vi "add parameter indicies controls.vi"(8 "error in":errorcluster, 9 "Channels to create":T1[](array[typedef]), 10 "class path":path, 11 "Application in":refnum<vi>) -> (0 "error out":errorcluster, 2 "Disable Channel Group?":bool[](array[boolean]))   [LabVIEW 2013, in "FixedChannelTBModuleDecideFeatures.lvclass"]
uses:
  FixedChannelTBModuleDecideFeatures.lvclass
  channel configuration.ctl
  <vilib>/NI/Tag Bus Module Framework/channel/channel classification.ctl
  <vilib>/NI/Tag Bus/tag/Data Type.ctl
  <vilib>/Utility/traverseref.llb/TRef TravTarget.ctl
  <vilib>/NI/Tag Bus Module Framework/channel/TBM channel.lvclass
  <vilib>/Utility/traverseref.llb/VI Scripting - Traverse.lvlib
  <vilib>/NI/Tag Bus/tag/tag descriptor.lvclass
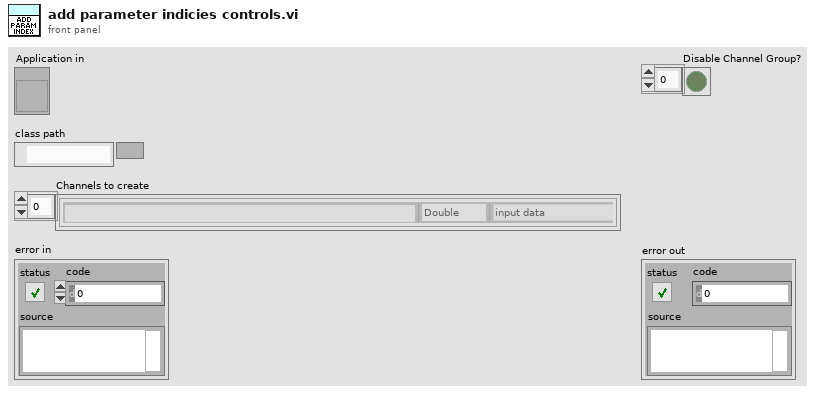
[diagram p1: front panel]
types:
  T1 = typedef "FixedChannelTBModuleDecideFeatures.lvclass/channel configuration.ctl" = cluster{"Name":string, "channel classification":T2, "data type":T3}
  T2 = typedef "TBM channel.lvclass/channel classification.ctl" = enum16{"input data", "output data", "processing parameter", "processing result"}
  T3 = typedef "tag bus.lvlib/tag descriptor.lvclass/Data Type.ctl" = enum16{"Double", "Single", "I64", "I32", "I16", "I8", "U64", "U32", "U16", "U8", "Boolean", "String", "Array of Double", "Array of Single", "Array of I64", "Array of I32", "Array of I16", "Array of I8", "Array of U64", "Array of U32", "Array of U16", "Array of U8", "Array of Boolean", "Array of String"}
  T4 = typedef "TRef TravTarget.ctl" = enum16{"FP", "BD", "Other"}
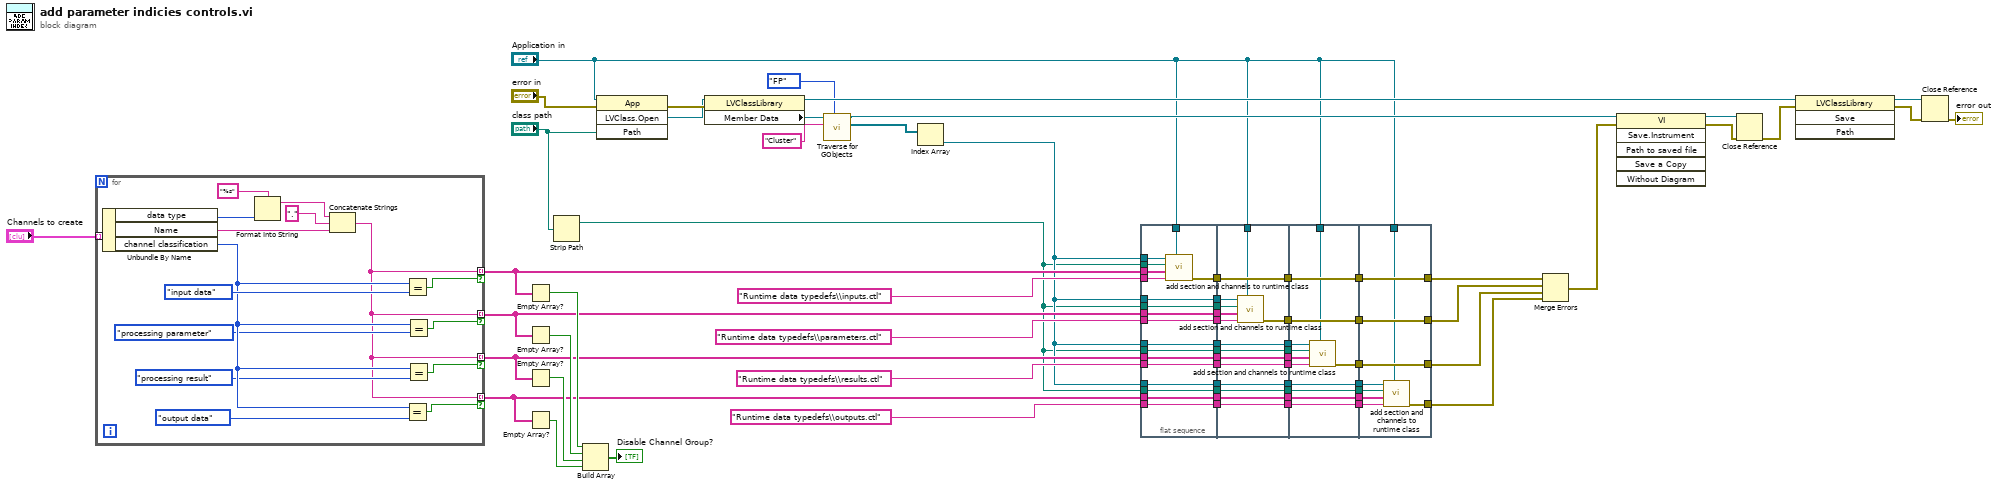
[diagram p0: block diagram]
diagram:
  n1 = for {
    tunnel: "Channels to create" -> [w84] mode=indexing
    tunnel: [w70] -> w51 mode=indexing if=w82
    tunnel: [w70] -> w47 mode=indexing if=w81
    tunnel: [w70] -> w37 mode=indexing if=w79
    tunnel: [w70] -> w25 mode=indexing if=w80
    n2 = Unbundle By Name(w84) -> ("data type"=w74:T3, "Name"=w72:string, "channel classification"=w78:T2)
    n3 = Format Into String(format string="%s", w74) -> (resulting string=w73:string)  [unwired: 2 in, 1 out]
    n4 = Concatenate Strings(w73, "." ("string"), w72) -> (w70:string)
    n5 = Equal?(x=w78, y=channel_classification."output data" ("x")) -> (x = y?=w80:bool)
    n6 = Equal?(x=w78, y=channel_classification."input data" ("x")) -> (x = y?=w82:bool)
    n7 = Equal?(x=w78, y=channel_classification."processing parameter" ("x")) -> (x = y?=w81:bool)
    n8 = Equal?(x=w78, y=channel_classification."processing result" ("x")) -> (x = y?=w79:bool)
  }
  n9 = Empty Array?(array=w51) -> (empty?=w56:bool)
  n10 = Empty Array?(array=w47) -> (empty?=w55:bool)
  n11 = Empty Array?(array=w37) -> (empty?=w54:bool)
  n12 = Empty Array?(array=w25) -> (empty?=w53:bool)
  n13 = Strip Path(path="class path") -> (stripped path=w26:path)  [unwired: 1 out]
  n14 = Build Array(w56, w55, w54, w53) -> (→"Disable Channel Group?":bool[])
  n15 = invoke class="App" method="LVClass.Open"(reference="Application in", error in="error in", "Path"="class path") -> (error out=w68:errorcluster, "LVClass.Open"=w2:refnum<vi>)  [unwired: 1 in, 2 out]
  n16 = property class="LVClassLibrary"(reference=w2, error in=w68) -> (reference out=w65:refnum<vi>, "Member Data"=w3:refnum<vi>)  [unwired: 1 out]
  n17 = call <vilib>:"Traverse for GObjects.vi"("Traverse Target"=TRef_TravTarget."FP", "Class Name"="Cluster", "VI Refnum"=w3) -> ("References"=w4:refnum<vi>[], "dup VI Refnum"=w7:refnum<vi>)  [unwired: 5 in, 2 out]
  n18 = Index Array(array=w4) -> (element=w30:refnum<vi>)  [unwired: 1 in]
  n19 = flat-sequence {
    tunnel: w51 -> [w102]
    tunnel: "Runtime data typedefs\\inputs.ctl" ("name or relative path") -> [w101]
    tunnel: w26 -> [w100]
    tunnel: w30 -> [w86]
    tunnel: w30 -> [w99]
    tunnel: [w99] -> w49
    tunnel: [w98] -> w48
    tunnel: w26 -> [w98]
    tunnel: w47 -> [w97]
    tunnel: [w97] -> w46
    tunnel: [w96] -> w45
    tunnel: "Runtime data typedefs\\parameters.ctl" ("name or relative path") -> [w96]
    tunnel: [w95] -> w42
    tunnel: w30 -> [w95]
    tunnel: [w94] -> w40
    tunnel: w26 -> [w94]
    tunnel: [w93] -> w38
    tunnel: w37 -> [w93]
    tunnel: "Runtime data typedefs\\results.ctl" ("name or relative path") -> [w92]
    tunnel: [w92] -> w34
    tunnel: [w91] -> w31
    tunnel: w30 -> [w91]
    tunnel: [w90] -> w27
    tunnel: w26 -> [w90]
    tunnel: w25 -> [w89]
    tunnel: [w89] -> w24
    tunnel: [w88] -> w19
    tunnel: "Runtime data typedefs\\outputs.ctl" ("name or relative path") -> [w88]
    tunnel: [w87] -> w14
    tunnel: "Application in" -> [w85]
    tunnel: w49 -> [w117]
    tunnel: w48 -> [w116]
    tunnel: w46 -> [w115]
    tunnel: w45 -> [w114]
    tunnel: [w113] -> w43
    tunnel: w42 -> [w113]
    tunnel: [w112] -> w41
    tunnel: w40 -> [w112]
    tunnel: [w111] -> w39
    tunnel: w38 -> [w111]
    tunnel: [w110] -> w35
    tunnel: w34 -> [w110]
    tunnel: [w109] -> w32
    tunnel: w31 -> [w109]
    tunnel: [w108] -> w28
    tunnel: w27 -> [w108]
    tunnel: w24 -> [w107]
    tunnel: [w107] -> w23
    tunnel: [w106] -> w20
    tunnel: w19 -> [w106]
    tunnel: [w105] -> w15
    tunnel: w14 -> [w105]
    tunnel: [w104] -> w12
    tunnel: "Application in" -> [w103]
    tunnel: w43 -> [w129]
    tunnel: w41 -> [w128]
    tunnel: w39 -> [w127]
    tunnel: w35 -> [w126]
    tunnel: [w125] -> w33
    tunnel: w32 -> [w125]
    tunnel: [w124] -> w29
    tunnel: w28 -> [w124]
    tunnel: w23 -> [w123]
    tunnel: [w123] -> w22
    tunnel: [w122] -> w21
    tunnel: w20 -> [w122]
    tunnel: [w121] -> w16
    tunnel: w15 -> [w121]
    tunnel: [w120] -> w13
    tunnel: w12 -> [w120]
    tunnel: [w119] -> w11
    tunnel: "Application in" -> [w118]
    tunnel: w33 -> [w138]
    tunnel: w29 -> [w137]
    tunnel: w22 -> [w136]
    tunnel: w21 -> [w135]
    tunnel: [w134] -> w17
    tunnel: w16 -> [w134]
    tunnel: [w133] -> w10
    tunnel: w13 -> [w133]
    tunnel: [w132] -> w9
    tunnel: w11 -> [w132]
    tunnel: [w131] -> w8
    tunnel: "Application in" -> [w130]
    frame #0 {
      n20 = call "add section and channels to runtime class.vi"("Application in"=w85, "Typedef relative path"=w101, "channels"=w102, "class base path"=w100, "class control ref"=w86) -> ("error out"=w87:errorcluster)  [unwired: 6 in]
    }
    frame #1 {
      n21 = call "add section and channels to runtime class.vi"("Application in"=w103, "Typedef relative path"=w114, "channels"=w115, "class base path"=w116, "class control ref"=w117) -> ("error out"=w104:errorcluster)  [unwired: 6 in]
    }
    frame #2 {
      n22 = call "add section and channels to runtime class.vi"("Application in"=w118, "Typedef relative path"=w126, "channels"=w127, "class base path"=w128, "class control ref"=w129) -> ("error out"=w119:errorcluster)  [unwired: 6 in]
    }
    frame #3 {
      n23 = call "add section and channels to runtime class.vi"("Application in"=w130, "Typedef relative path"=w135, "channels"=w136, "class base path"=w137, "class control ref"=w138) -> ("error out"=w131:errorcluster)  [unwired: 6 in]
    }
  }
  n24 = Merge Errors(w17, w10, w9, w8) -> (w57:errorcluster)
  n25 = invoke class="VI" method="Save.Instrument"(reference=w7, error in=w57) -> (reference out=w60:refnum<vi>, error out=w61:errorcluster)  [unwired: 4 in, 4 out]
  n26 = Close Reference(reference=w60, error in (no error)=w61) -> (error out=w62:errorcluster)
  n27 = invoke class="LVClassLibrary" method="Save"(reference=w65, error in=w62) -> (reference out=w64:refnum<vi>, error out=w63:errorcluster)  [unwired: 2 in, 2 out]
  n28 = Close Reference(reference=w64, error in (no error)=w63) -> (error out=→"error out":errorcluster)
